vi "AB_Convert_To_ExportedVI.vi"(8 "error in (no error)":errorcluster, 10 "Source in":refnum<class "AB_Source.lvclass">, 11 "Build in":refnum<class "AB_Build.lvclass">) -> (0 "error out":errorcluster, 3 "Exported VI out":refnum<class "AB_Source_VI.lvclass">)   [LabVIEW 2020]
uses:
  <vilib>/AppBuilder/AB_Classes/Build/AB_Build.lvclass
  <vilib>/AppBuilder/AB_Classes/Source/AB_Source.lvclass
  <vilib>/AppBuilder/AB_Classes/Source/VI/AB_Source_VI.lvclass
  e:/builds/penguin/labview/branches/2020/dev/dist/vi.lib/AppBuilder/AB_Classes/Source/AB_Source.lvclass
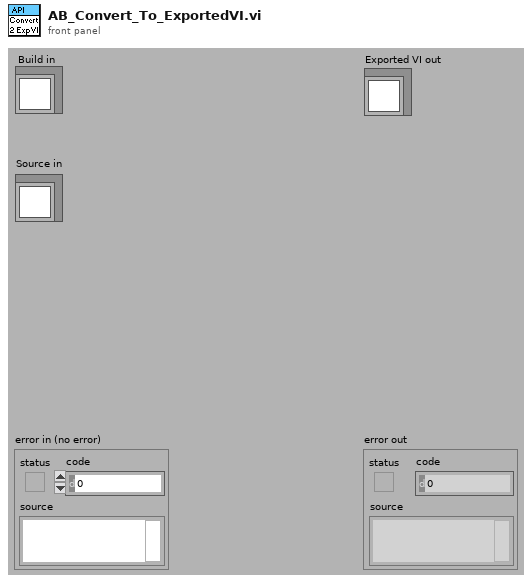
[diagram p1: front panel]
types:
  T1 = typedef "AB_Source.ctl" = cluster{"path":path, "itemID":string, "parentIndex":i32, "sourceInclusion":T2, "destinationIndex":i32, "properties":T3[], "newName":string, "lvfile":bool, "valid":bool, "eng_inBuild":bool, "eng_isNonVILink":bool, "Amalgamation":bool, "Amalgamation Piece":bool, "eng_delimitedName":string, "preventRename":bool}
  T2 = typedef "AB_Source_Inclusion.ctl" = enum16{"IncludeIfReferenced", "Include", "Exclude", "TopLevel"}
  T3 = typedef "AB_Source_Properties.ctl" = cluster{"sourcePropertyType":T4, "value":variant}
  T4 = typedef "AB_Source_Property_Type.ctl" = enum16{"Remove block diagram", "Remove front panel", "Password", "Window has title bar", "Show menu bar", "Show vertical scroll bar", "Show horizontal scroll bar", "Show toolbar", "Show Abort button", "Show fp when called", "Window behavior", "Allow user to close window", "Window run-time position", "Run when opened", "Allow debugging", "Auto error handling", "Generate guard code", "Use stack variables", "Expression folding", "Integer only", "Inline subVI"}
  T5 = typedef "AB_Source_VI.ctl" = cluster{"standardVI":bool, "dynamicDispatch":bool, "LLBtopLevel":bool, "privateDataControl":bool, "eng_hasNonVILinks":bool, "eng_reference":refnum<vi>, "eng_saveLevel":u32}
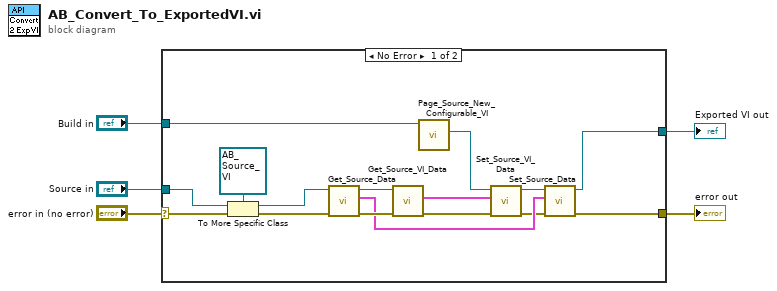
[diagram p0: block diagram]
diagram:
  n1 = case shown="No Error" "error in (no error)" {
    selector: "error in (no error)" -> [w8 w22]
    tunnel: [w6 w22] -> w4
    tunnel: "Source in" -> [w10 _]
    tunnel: "Build in" -> [w9 _]
    tunnel: [w7 _] -> w1
    frame No Error {
      n2 = To More Specific Class(target class=refnum<class "AB_Source_VI.lvclass"> refnum ("AB_Source_VI.lvclass"), reference=w10, error in=w8) -> (specific class reference=w20:refnum<class "AB_Source_VI.lvclass">, error out=w19:errorcluster)
      n3 = call <vilib>:"Get_Source_Data.vi"("error in (no error)"=w19, "Class in"=w20) -> ("error out"=w17:errorcluster, "data"=w13:T1, "Class out"=w18:refnum<class "AB_Source_VI.lvclass">)  [unwired: 7 out]
      n4 = call <vilib>:"Get_Source_VI_Data.vi"("error in (no error)"=w17, "Class in"=w18) -> ("error out"=w15:errorcluster, "data"=w16:T5)  [unwired: 8 out]
      n5 = call-dynamic "Page_Source_New_Configurable_VI.vi"("AB_Build in"=w9) -> ("AB_Source_VI out"=w11:refnum<class "AB_Source_VI.lvclass">)  [unwired: 1 in, 9 out]
      n6 = call <vilib>:"Set_Source_VI_Data.vi"("error in (no error)"=w15, "data"=w16, "Class in"=w11) -> ("error out"=w12:errorcluster, "Class out"=w14:refnum<class "AB_Source_VI.lvclass">)  [unwired: 7 out]
      n7 = call <vilib>:"Set_Source_Data.vi"("error in (no error)"=w12, "data"=w13, "Class in"=w14) -> ("error out"=w6:errorcluster, "Class out"=w7:refnum<class "AB_Source_VI.lvclass">)  [unwired: 7 out]
    }
    frame Error {
    }
  }
  "error out" <- w4
  "Exported VI out" <- w1
